vi "Ctor.vi"(7 "I2C Channel":u8, 8 "error in (no error)":errorcluster, 10 "Address":T8=40 items=["0x28"=40, "0x29"=41], 11 "LINX Resource":T2) -> (0 "error out":errorcluster, 2 "IDs":T1, 3 "BNO055 out":refnum<class "BNO055.lvclass">)   [LabVIEW 2020, in "BNO055.lvlib" / "BNO055.lvclass"]
uses:
  BNO055.lvclass
  Address.ctl
  <vilib>/MakerHub/LINX/Private/Type Defs/LINX Ref.ctl
  <vilib>/MakerHub/LINX/Private/Type Defs/Platform.ctl
  <vilib>/MakerHub/LINX/Private/Type Defs/Interface.ctl
  <vilib>/MakerHub/LINX/Private/Device/Type Defs/LINX Device Config.ctl
  <vilib>/MakerHub/LINX/Private/Device/Type Defs/TCP Config.ctl
  <vilib>/MakerHub/LINX/Private/Device/Type Defs/Channels.ctl
  IDs.ctl
  Ref Data.ctl
  Operating Mode.ctl
  BNO055.lvclass/BNO055.ctl
  <vilib>/MakerHub/LINX/LMH-LINX.lvlib
  <vilib>/MakerHub/LINX/Private/Device/Device.lvlib
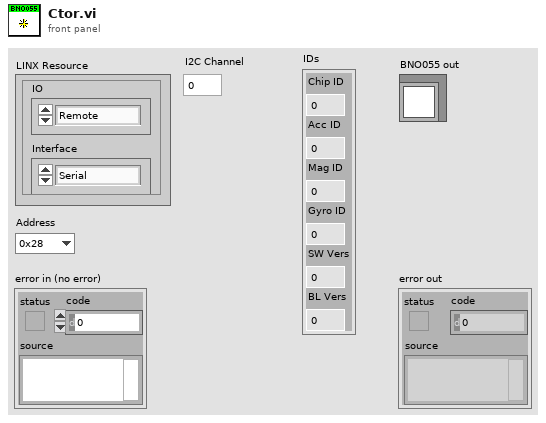
[diagram p1: front panel]
types:
  T1 = typedef "BNO055.lvlib/BNO055.lvclass/IDs.ctl" = cluster{"Chip ID":u8, "Acc ID":u8, "Mag ID":u8, "Gyro ID":u8, "SW Vers":u16, "BL Vers":u8}
  T2 = typedef "LMH-LINX.lvlib/LINX Ref.ctl" = cluster{"IO":T3, "Interface":T4, "LINX Device Config":T5}
  T3 = typedef "LMH-LINX.lvlib/Platform.ctl" = enum16{"Remote", "Local"}
  T4 = typedef "LMH-LINX.lvlib/Interface.ctl" = enum16{"Serial", "TCP"}
  T5 = typedef "LMH-LINX.lvlib/Device.lvlib/LINX Device Config.ctl" = cluster{"Interface":T4, "COM Port":refnum<visa-resource-name>, "TCP Configuration":T6, "Device Family":u8, "Device ID":u8, "Device Name":string, "TCP Ref":refnum<k5>, "Channels":T7}
  T6 = typedef "LMH-LINX.lvlib/Device.lvlib/TCP Config.ctl" = cluster{"IP Address":string, "Port":u16}
  T7 = typedef "LMH-LINX.lvlib/Channels.ctl" = cluster{"DI":u8[], "DO":u8[], "AI":u8[], "AO":u8[], "PWM":u8[], "QE":u8[], "UART":u8[], "I2C 2":u8[], "SPI":u8[], "CAN":u8[], "Servo":u8[], "AI Ref (V)":dbl, "AI Resolution (Bits)":u8, "AO Ref (V)":dbl, "AO Resolution (Bits)":u8}
  T8 = typedef "BNO055.lvlib/BNO055.lvclass/Address.ctl" = u8
  T9 = typedef "BNO055.lvlib/BNO055.lvclass/Ref Data.ctl" = cluster{"Operating Mode":T10}
  T10 = typedef "BNO055.lvlib/BNO055.lvclass/Operating Mode.ctl" = enum8{"Config", "Acc Only", "Mag Only", "Gyr Only", "Acc Mag", "Acc Gyr", "Mag Gyr", "AccMagGyr", "IMU", "Compass", "Mag4Gyr", "NDOF FMC Off", "NDOF"}
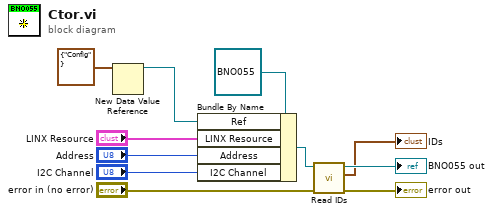
[diagram p0: block diagram]
diagram:
  n1 = New Data Value Reference(data value=T9 {"Operating Mode"=enum."Config"} ("Ref Data")) -> (data value reference=w8:refnum<data-value>)  [unwired: 1 in, 1 out]
  n2 = Bundle By Name(cluster=refnum<class "BNO055.lvclass"> refnum ("BNO055 out"), "Ref"=w8, "LINX Resource"="LINX Resource", "Address"="Address", "I2C Channel"="I2C Channel") -> (w4:refnum<class "BNO055.lvclass">)
  n3 = call "Read IDs.vi"("error in (no error)"="error in (no error)", "BNO055 in"=w4) -> ("error out"=→"error out":errorcluster, "IDs"=→"IDs":T1, "BNO055 out"=→"BNO055 out":refnum<class "BNO055.lvclass">)  [unwired: 7 in]
